vi "VSG25_RampSweep.vi"(0 "Device Handle In":i32, 1 "Run as Subpanel":bool, 2 "RampSweep Cluster In":T1 {"Start Hz" items=["Hz", "kHz", "MHz", "GHz"]; "Stop Hz" items=["Hz", "kHz", "MHz", "GHz"]; "Step Hz" items=["Hz", "kHz", "MHz", "GHz"]}, 3 "Error In":errorcluster) -> (5 "Device Handle Out":i32, 6 "RampSweep Cluster Out":T1 {"Start Hz" items=["Hz", "kHz", "MHz", "GHz"]; "Stop Hz" items=["Hz", "kHz", "MHz", "GHz"]; "Step Hz" items=["Hz", "kHz", "MHz", "GHz"]}, 7 "Error Out":errorcluster)   [LabVIEW 2014]
uses:
  Frequency Hertz.ctl
  RampSweep Cluster.ctl
  sg_lib/VSG25A.lvlib
panel:
  out "Sweep Time":dbl
  out "Frequency Span":dbl
  in  "Dwell Time (mS)":dbl
  in  "Stop":bool
  out "Device Selected":bool
  in  "Step Hz":T2 items=["Hz", "kHz", "MHz", "GHz"]
  in  "Step Frequency":dbl
  in  "Stop Hz":T2 items=["Hz", "kHz", "MHz", "GHz"]
  in  "Stop Frequency":dbl
  in  "RF On":bool
  in  "Start Hz":T2 items=["Hz", "kHz", "MHz", "GHz"]
  in  "Amplitude (dBm)":dbl
  in  "Start Frequency":dbl
  # "Ramp Sweep"
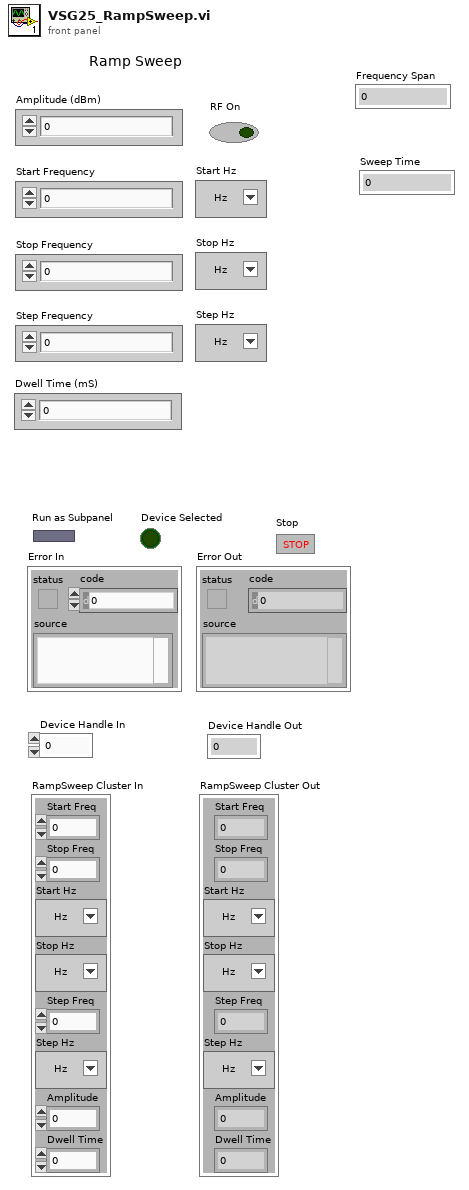
[diagram p1: front panel]
types:
  T1 = typedef "RampSweep Cluster.ctl" = cluster{"Start Freq":dbl, "Stop Freq":dbl, "Start Hz":T2, "Stop Hz":T2, "Step Freq":dbl, "Step Hz":T2, "Amplitude":dbl, "Dwell Time":dbl}
  T2 = typedef "Frequency Hertz.ctl" = u16
  T3 = enum16{"Init", "Proc Events", "Write VSG25", "Exit"}
  T4 = enum32{"Bad", "Idle", "Run top level", "Running"}
  T5 = enum16{"Check Amplitude", "Check Start Freq", "Check Stop Freq", "Check Step Freq", "Check Dwell Time", "Calc Freq Span", "Calc Sweep Time", "Stop RF", "Set Freq And Amp", "Set Sweep", "Finish", ""}
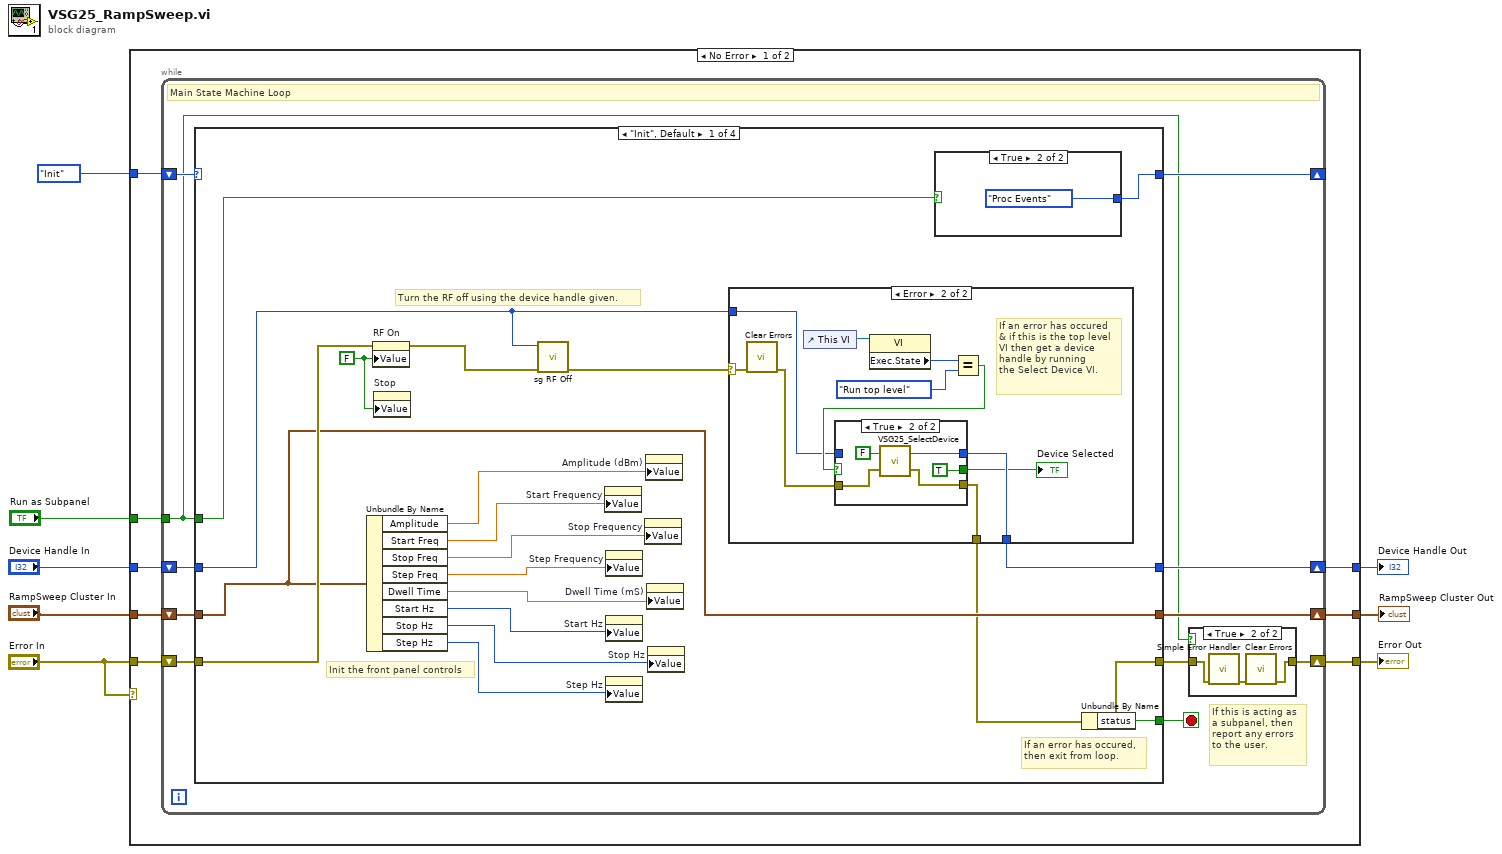
[diagram p0: block diagram]
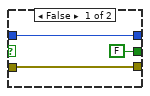
[diagram p4: hidden frame]
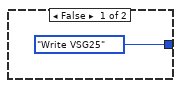
[diagram p5: hidden frame]
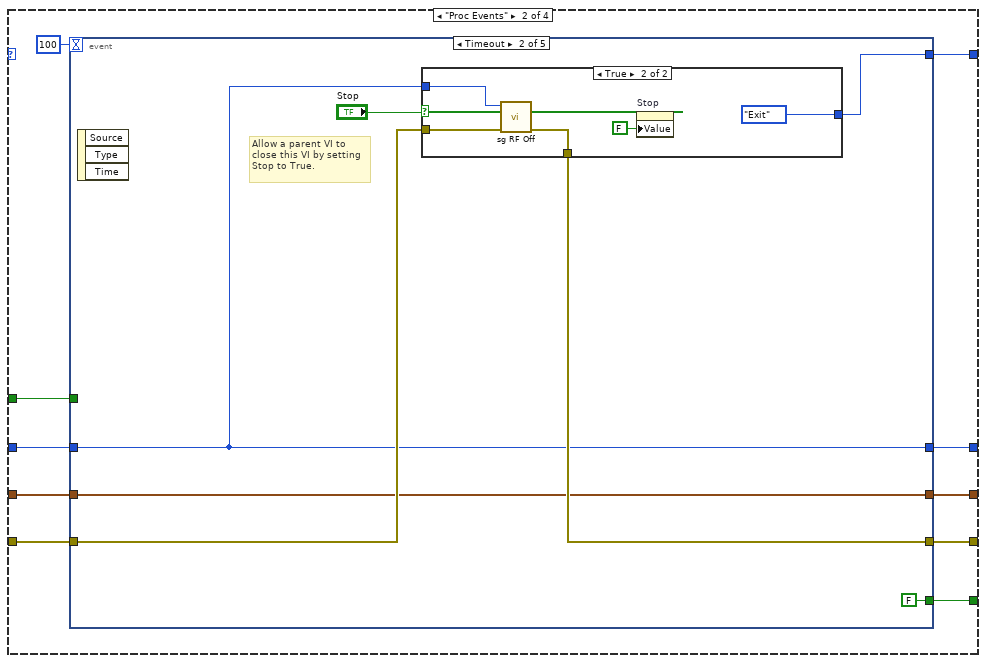
[diagram p6: hidden frame]
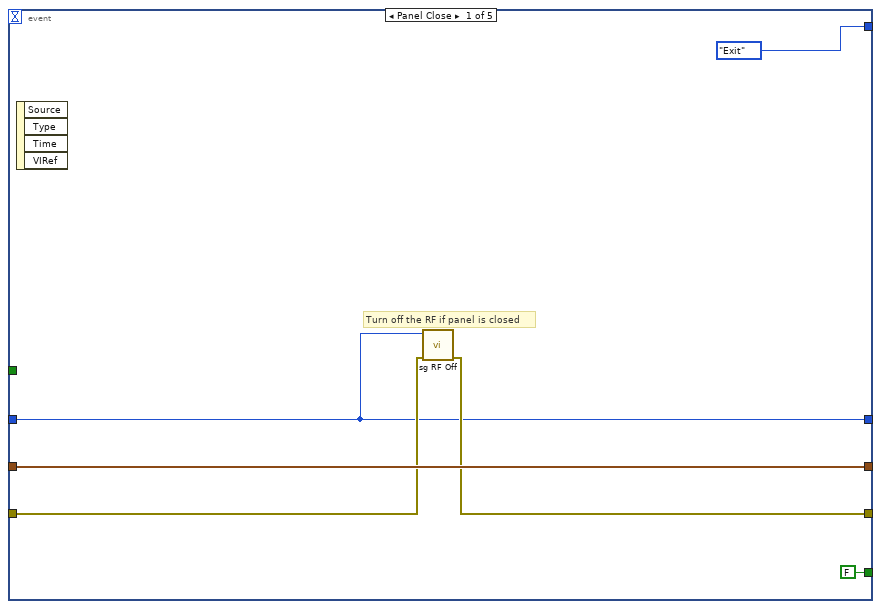
[diagram p7: hidden frame]
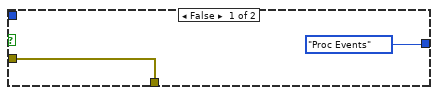
[diagram p8: hidden frame]
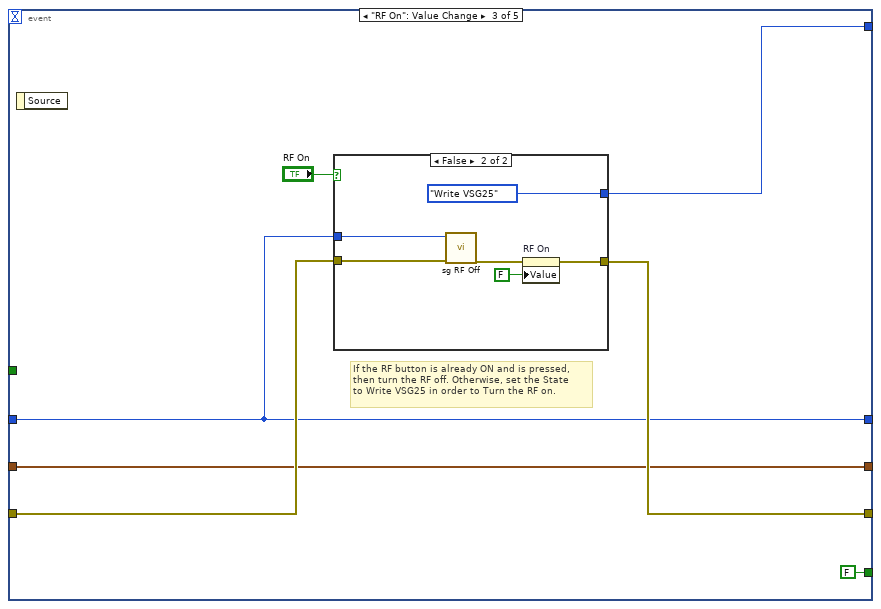
[diagram p9: hidden frame]
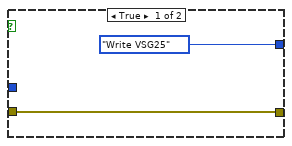
[diagram p10: hidden frame]
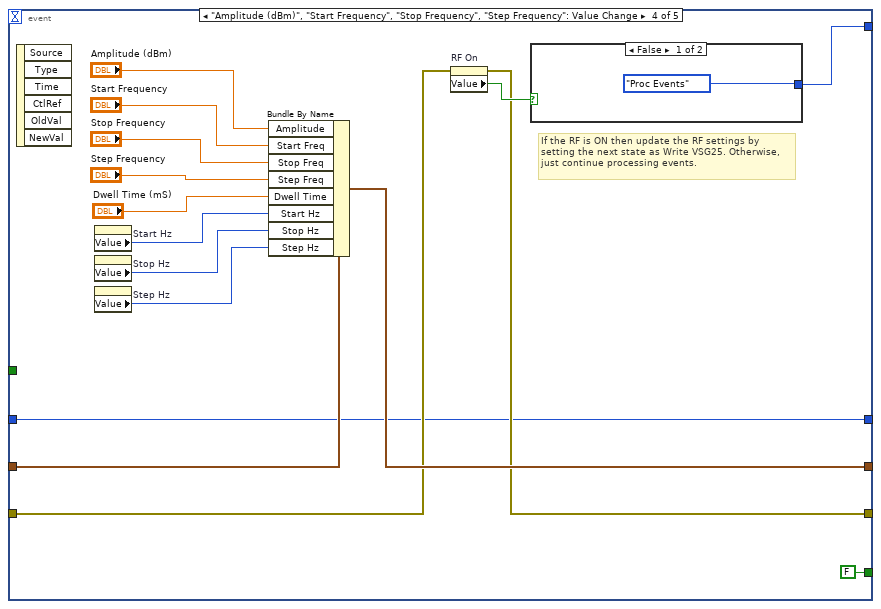
[diagram p11: hidden frame]
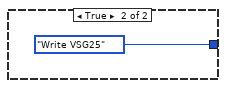
[diagram p12: hidden frame]
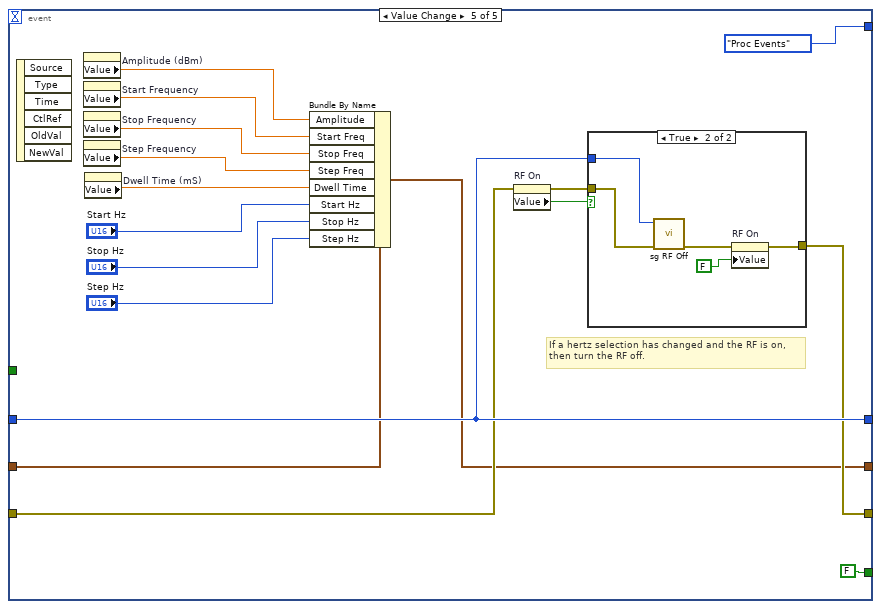
[diagram p13: hidden frame]
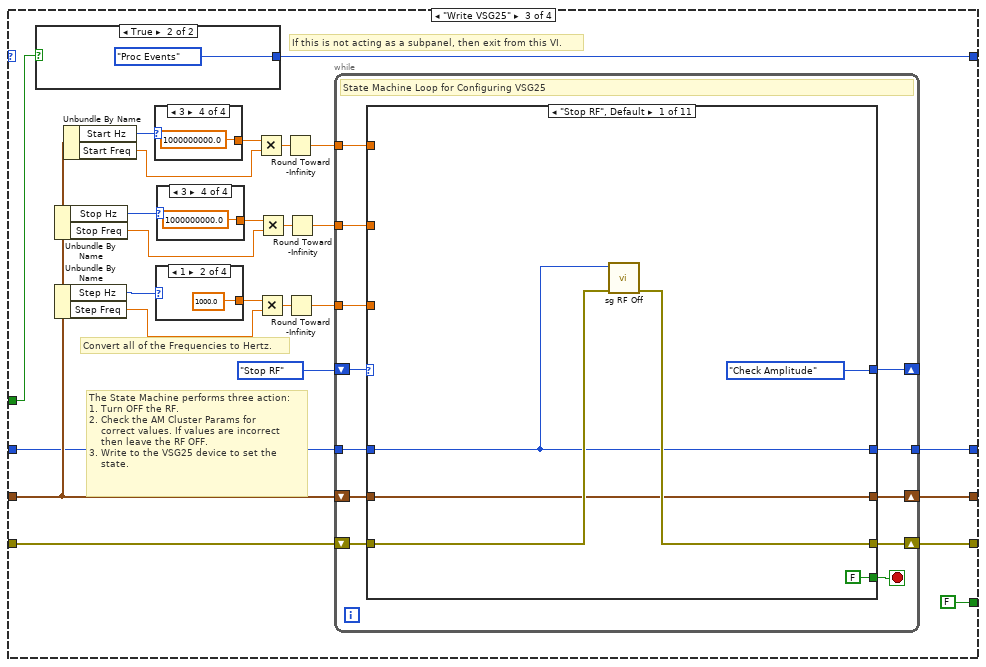
[diagram p15: hidden frame]
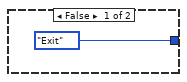
[diagram p16: hidden frame]
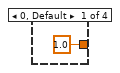
[diagram p17: hidden frame]
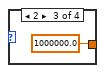
[diagram p18: hidden frame]
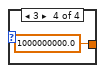
[diagram p19: hidden frame]
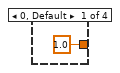
[diagram p20: hidden frame]
diagram:
  n1 = case shown="No Error" "Error In" {
    tunnel: "Error In" -> [w12 w376]
    tunnel: T3."Init" -> [w16 _]
    tunnel: "Run as Subpanel" -> [w15 _]
    tunnel: "Device Handle In" -> [w14 w374]
    tunnel: "RampSweep Cluster In" -> [w13 w375]
    tunnel: [w11 w376] -> w4
    tunnel: [w10 w375] -> w1
    tunnel: [w9 w374] -> w3
    frame No Error {
      n2 = while {
        shift-right: [w26] -> _
        shift-left: w16 -> [w27]
        tunnel: w15 -> [w17]
        shift-right: [w18] -> w11
        shift-left: w12 -> [w23]
        shift-right: [w21] -> w10
        shift-left: w13 -> [w24]
        shift-right: [w20] -> w9
        shift-left: w14 -> [w25]
        stop <- w22 stop-if-true
        # "If this is acting as \na subpanel, then\nreport any errors\nto the user."
        # "Main State Machine Loop"
        n3 = case shown="\"Init\", Default" w27 {
          selector: w27 -> [_ _ _ w369]
          tunnel: [w43 w75 w161 w369] -> w26
          tunnel: w17 -> [w46 w79 w160 _]
          tunnel: w25 -> [w37 w80 w166 w364]
          tunnel: w24 -> [w44 w81 w167 w365]
          tunnel: w23 -> [w45 w82 w171 w366]
          tunnel: [w42 w76 FALSE TRUE] -> w22
          tunnel: [w38 w74 w165 w367] -> w19
          tunnel: [w44 w78 w164 w365] -> w21
          tunnel: [w39 w77 w163 w364] -> w20
          frame "Init", Default {
            w36 = FALSE ("RF On")
            # "Init the front panel controls"
            # "Turn the RF off using the device handle given."
            # "If an error has occured,\nthen exit from loop."
            n4 = Unbundle By Name(w44) -> ("Amplitude"=w50:dbl, "Start Freq"=w49:dbl, "Stop Freq"=w48:dbl, "Step Freq"=w47:dbl, "Dwell Time"=w32:dbl, "Start Hz"=w35:T2, "Stop Hz"=w34:T2, "Step Hz"=w33:T2)
            n5 = property on="RF On" class="Bool (strict)"(error in=w45, "Value"=w36) -> (error out=w41:errorcluster)  [unwired: 1 in, 1 out]
            n6 = property on="Stop" class="Bool (strict)"("Value"=w36) -> ()  [unwired: 2 in, 2 out]
            n7 = call "sg RF Off.vi"("error in (no error)"=w41, "device"=w37) -> ("error out"=w40:errorcluster)  [unwired: 8 in, 1 out]
            n8 = property on="Start Frequency" class="DigNum (strict)"("Value"=w49) -> ()  [unwired: 2 in, 2 out]
            n9 = property on="Step Frequency" class="DigNum (strict)"("Value"=w47) -> ()  [unwired: 2 in, 2 out]
            n10 = property on="Start Hz" class="Ring (strict)"("Value"=w35) -> ()  [unwired: 2 in, 2 out]
            n11 = property on="Step Hz" class="Ring (strict)"("Value"=w33) -> ()  [unwired: 2 in, 2 out]
            n12 = property on="Stop Frequency" class="DigNum (strict)"("Value"=w48) -> ()  [unwired: 2 in, 2 out]
            n13 = property on="Amplitude (dBm)" class="DigNum (strict)"("Value"=w50) -> ()  [unwired: 2 in, 2 out]
            n14 = property on="Dwell Time (mS)" class="DigNum (strict)"("Value"=w32) -> ()  [unwired: 2 in, 2 out]
            n15 = property on="Stop Hz" class="Ring (strict)"("Value"=w34) -> ()  [unwired: 2 in, 2 out]
            n16 = case shown="Error" w40 {
              selector: w40 -> [w51 w58]
              tunnel: [w52 w56] -> w39
              tunnel: [w51 w55] -> w38
              tunnel: w37 -> [w52 w54]
              frame No Error {
              }
              frame Error {
                # "If an error has occured\n& if this is the top level\nVI then get a device\nhandle by running \nthe Select Device VI."
                n17 = call <vilib>:"Clear Errors.vi"("error in (no error)"=w58) -> ("error out"=w57:errorcluster)  [unwired: 5 in, 1 out]
                n18 = control-ref of="This VI"() -> (w62:refnum<vi>)
                n19 = property class="VI"(reference=w62) -> ("Exec.State"=w61:T4)  [unwired: 1 in, 2 out]
                n20 = Equal?(x=w61, y=T4."Run top level" ("Execution:State 2")) -> (x = y?=w59:bool)
                n21 = case shown="True" w59 {
                  tunnel: [w65 w70] -> w56
                  tunnel: w54 -> [w65 _]
                  tunnel: w57 -> [w64 w68]
                  tunnel: [w64 w67] -> w55
                  tunnel: [FALSE TRUE] -> w53
                  frame False {
                  }
                  frame True {
                    n22 = call "VSG25_SelectDevice.vi"("ErrorIn"=w68, "AutoSel"=FALSE) -> ("ErrorOut"=w67:errorcluster, "deviceHandle"=w70:i32)
                  }
                }
                "Device Selected" <- w53
              }
            }
            n23 = case shown="True" w46 {
              tunnel: [T3."Write VSG25" T3."Proc Events"] -> w43
              frame False {
              }
              frame True {
              }
            }
            n24 = Unbundle By Name(w38) -> ("status"=w42:bool)
          }
          frame "Proc Events" {
            n25 = event shown="[1] Timeout" {
              selector: _ -> [_ _ _ _ _]
              dyn-events: _ -> [_ _ _ _ _]
              timeout: 100 -> [_ _ _ _ _]
              tunnel: w82 -> [w85 w92 w108 w125 w148]
              tunnel: w81 -> [w86 w90 w106 w133 w147]
              tunnel: w80 -> [w83 w89 w105 w123 w150]
              tunnel: w79 -> [_ _ _ _ _]
              tunnel: [w84 w91 w107 w124 w149] -> w74
              tunnel: [w86 w90 w106 w132 w146] -> w78
              tunnel: [w83 w89 w105 w123 w150] -> w77
              tunnel: [FALSE FALSE FALSE FALSE FALSE] -> w76
              tunnel: [T3."Exit" w93 w104 w126 T3."Proc Events"] -> w75
              event Panel Close {
                # "Turn off the RF if panel is closed"
                n26 = event-data() -> ()  [unwired: 1 in, 4 out]
                n27 = call "sg RF Off.vi"("error in (no error)"=w85, "device"=w83) -> ("error out"=w84:errorcluster)  [unwired: 8 in, 1 out]
              }
              event Timeout {
                # "Allow a parent VI to \nclose this VI by setting\nStop to True."
                n28 = event-data() -> ()  [unwired: 1 in, 3 out]
                n29 = case shown="True" "Stop" {
                  tunnel: [T3."Proc Events" T3."Exit"] -> w93
                  tunnel: w92 -> [w96 w101]
                  tunnel: [w96 w100] -> w91
                  tunnel: w89 -> [_ w99]
                  frame False {
                  }
                  frame True {
                    n30 = call "sg RF Off.vi"("error in (no error)"=w101, "device"=w99) -> ("error out"=w100:errorcluster)  [unwired: 8 in, 1 out]
                    n31 = property on="Stop" class="Bool (strict)"("Value"=FALSE ("Stop")) -> ()  [unwired: 2 in, 2 out]
                  }
                }
              }
              event "RF On": Value Change {
                # "If the RF button is already ON and is pressed, \nthen turn the RF off. Otherwise, set the State\nto Write VSG25 in order to Turn the RF on."
                n32 = event-data() -> ()  [unwired: 1 in, 1 out]
                n33 = case shown="False" "RF On" {
                  tunnel: [w110 w115] -> w107
                  tunnel: w108 -> [w110 w117]
                  tunnel: w105 -> [_ w116]
                  tunnel: [T3."Write VSG25" T3."Write VSG25"] -> w104
                  frame True {
                  }
                  frame False {
                    n34 = call "sg RF Off.vi"("error in (no error)"=w117, "device"=w116) -> ("error out"=w114:errorcluster)  [unwired: 8 in, 1 out]
                    n35 = property on="RF On" class="Bool (strict)"(error in=w114, "Value"=FALSE ("RF On")) -> (error out=w115:errorcluster)  [unwired: 1 in, 1 out]
                  }
                }
              }
              event "Amplitude (dBm)", "Start Frequency", "Stop Frequency", "Step Frequency": Value Change {
                # "If the RF is ON then update the RF settings by\nsetting the next state as Write VSG25. Otherwise,\njust continue processing events."
                n36 = event-data() -> ()  [unwired: 1 in, 6 out]
                n37 = property on="Start Hz" class="Ring (strict)"() -> ("Value"=w120:T2)  [unwired: 2 in, 2 out]
                n38 = property on="Stop Hz" class="Ring (strict)"() -> ("Value"=w119:T2)  [unwired: 2 in, 2 out]
                n39 = property on="Step Hz" class="Ring (strict)"() -> ("Value"=w118:T2)  [unwired: 2 in, 2 out]
                n40 = Bundle By Name(cluster=w133, "Amplitude"="Amplitude (dBm)", "Start Freq"="Start Frequency", "Stop Freq"="Stop Frequency", "Step Freq"="Step Frequency", "Dwell Time"="Dwell Time (mS)", "Start Hz"=w120, "Stop Hz"=w119, "Step Hz"=w118) -> (w132:T1)
                n41 = property on="RF On" class="Bool (strict)"(error in=w125) -> (error out=w124:errorcluster, "Value"=w127:bool)  [unwired: 1 in, 1 out]
                n42 = case shown="False" w127 {
                  tunnel: [T3."Proc Events" T3."Write VSG25"] -> w126
                  frame False {
                  }
                  frame True {
                  }
                }
              }
              event Value Change {
                # "If a hertz selection has changed and the RF is on,\nthen turn the RF off."
                n43 = event-data() -> ()  [unwired: 1 in, 6 out]
                n44 = property on="Amplitude (dBm)" class="DigNum (strict)"() -> ("Value"=w145:dbl)  [unwired: 2 in, 2 out]
                n45 = property on="Start Frequency" class="DigNum (strict)"() -> ("Value"=w144:dbl)  [unwired: 2 in, 2 out]
                n46 = property on="Stop Frequency" class="DigNum (strict)"() -> ("Value"=w143:dbl)  [unwired: 2 in, 2 out]
                n47 = property on="Step Frequency" class="DigNum (strict)"() -> ("Value"=w142:dbl)  [unwired: 2 in, 2 out]
                n48 = property on="Dwell Time (mS)" class="DigNum (strict)"() -> ("Value"=w139:dbl)  [unwired: 2 in, 2 out]
                n49 = Bundle By Name(cluster=w147, "Amplitude"=w145, "Start Freq"=w144, "Stop Freq"=w143, "Step Freq"=w142, "Dwell Time"=w139, "Start Hz"="Start Hz", "Stop Hz"="Stop Hz", "Step Hz"="Step Hz") -> (w146:T1)
                n50 = property on="RF On" class="Bool (strict)"(error in=w148) -> (error out=w152:errorcluster, "Value"=w151:bool)  [unwired: 1 in, 1 out]
                n51 = case shown="True" w151 {
                  tunnel: [w153 w154] -> w149
                  tunnel: w152 -> [w153 w158]
                  tunnel: w150 -> [_ w157]
                  frame False {
                  }
                  frame True {
                    n52 = call "sg RF Off.vi"("error in (no error)"=w158, "device"=w157) -> ("error out"=w155:errorcluster)  [unwired: 8 in, 1 out]
                    n53 = property on="RF On" class="Bool (strict)"(error in=w155, "Value"=FALSE ("RF On")) -> (error out=w154:errorcluster)  [unwired: 1 in, 1 out]
                  }
                }
              }
            }
          }
          frame "Write VSG25" {
            # "If this is not acting as a subpanel, then exit from this VI."
            # "Convert all of the Frequencies to Hertz."
            # "The State Machine performs three action:\n1. Turn OFF the RF.\n2. Check the AM Cluster Params for \n    correct values. If values are incorrect\n    then leave the RF OFF.\n3. Write to the VSG25 device to set the\n    state."
            n54 = case shown="True" w160 {
              tunnel: [T3."Exit" T3."Proc Events"] -> w161
              frame False {
              }
              frame True {
              }
            }
            n55 = Unbundle By Name(w167) -> ("Stop Hz"=w177:T2, "Stop Freq"=w179:dbl)
            n56 = Unbundle By Name(w167) -> ("Step Hz"=w173:T2, "Step Freq"=w175:dbl)
            n57 = Unbundle By Name(w167) -> ("Start Hz"=w182:T2, "Start Freq"=w180:dbl)
            n58 = case shown="3" w182 {
              tunnel: [1.0 ("y") 1000.0 ("y") 1000000.0 ("y") 1000000000.0 ("y")] -> w181
              frame 0, Default {
              }
              frame 1 {
              }
              frame 2 {
              }
              frame 3 {
              }
            }
            n59 = case shown="1" w173 {
              tunnel: [1.0 ("y") 1000.0 ("y") 1000000.0 ("y") 1000000000.0 ("y")] -> w174
              frame 0, Default {
              }
              frame 1 {
              }
              frame 2 {
              }
              frame 3 {
              }
            }
            n60 = case shown="3" w177 {
              tunnel: [1.0 ("y") 1000.0 ("y") 1000000.0 ("y") 1000000000.0 ("y")] -> w178
              frame 0, Default {
              }
              frame 1 {
              }
              frame 2 {
              }
              frame 3 {
              }
            }
            n61 = Multiply(x=w181, y=w180) -> (x*y=w183:dbl)
            n62 = Multiply(x=w174, y=w175) -> (x*y=w172:dbl)
            n63 = Multiply(x=w178, y=w179) -> (x*y=w176:dbl)
            n64 = Round Toward -Infinity(1:w183) -> (0:w170:dbl)
            n65 = Round Toward -Infinity(1:w172) -> (0:w168:dbl)
            n66 = Round Toward -Infinity(1:w176) -> (0:w169:dbl)
            n67 = while {
              shift-right: [w194] -> _
              shift-left: T5."Stop RF" -> [w205]
              tunnel: w170 -> [w203]
              tunnel: w169 -> [w202]
              tunnel: w168 -> [w201]
              tunnel: w166 -> [w199]
              tunnel: [w196] -> w163
              shift-right: [w198] -> w165
              shift-left: w171 -> [w204]
              shift-right: [w197] -> w164
              shift-left: w167 -> [w200]
              stop <- w195 stop-if-true
              # "State Machine Loop for Configuring VSG25"
              n68 = case shown="\"Stop RF\", Default" w205 {
                selector: w205 -> [_ _ _ _ _ _ _ _ _ _ w354]
                tunnel: w204 -> [w211 w214 w252 w270 w288 w305 w317 w322 w340 w349 w351]
                tunnel: w203 -> [_ _ w242 _ _ _ w315 _ w332 _ _]
                tunnel: w202 -> [_ _ w244 w264 _ _ w314 _ _ _ _]
                tunnel: w201 -> [_ _ w243 _ w282 _ _ _ _ _ _]
                tunnel: w200 -> [w209 w218 w253 w272 w290 w303 w321 w323 w338 w347 w352]
                tunnel: w199 -> [w208 w216 w254 w271 w289 w302 w320 w330 w337 w346 w353]
                tunnel: [w210 w213 w251 w269 w287 w304 w317 w322 w339 w348 w351] -> w198
                tunnel: [w209 w217 w253 w272 w290 w303 w321 w323 w338 w347 w352] -> w197
                tunnel: [w208 w216 w254 w271 w289 w302 w320 w330 w337 w346 w353] -> w196
                tunnel: [FALSE FALSE FALSE FALSE FALSE FALSE FALSE FALSE FALSE FALSE TRUE] -> w195
                tunnel: [T5."Check Amplitude" w212 w256 w274 w292 w299 T5."Calc Sweep Time" T5."Set Freq And Amp" T5."Set Sweep" T5."Finish" w354] -> w194
                frame "Stop RF", Default {
                  n69 = call "sg RF Off.vi"("error in (no error)"=w211, "device"=w208) -> ("error out"=w210:errorcluster)  [unwired: 8 in, 1 out]
                }
                frame "Check Amplitude" {
                  n70 = Unbundle By Name(w218) -> ("Amplitude"=w224:dbl)
                  n71 = Less Or Equal?(x=w224, y=10.0) -> (x <= y?=w220:bool)
                  n72 = Greater Or Equal?(x=w224, y=-80.0) -> (x >= y?=w223:bool)
                  n73 = And(x=w220, y=w223) -> (x .and. y?=w219:bool)
                  n74 = case shown="True" w219 {
                    tunnel: w223 -> [w234 _]
                    tunnel: w224 -> [_ w239]
                    tunnel: w218 -> [w231 w238]
                    tunnel: [w230 w237] -> w217
                    tunnel: [T5."Finish" T5."Check Start Freq"] -> w212
                    tunnel: w214 -> [w228 w236]
                    tunnel: [w226 w236] -> w213
                    frame False {
                      n75 = Select(t=10.0, s=w234, f=-80.0) -> (s? t:f=w229:dbl)
                      n76 = Bundle By Name(cluster=w231, "Start Freq"=w229) -> (w230:T1)
                      n77 = property on="Amplitude (dBm)" class="DigNum (strict)"("Value"=w229) -> ()  [unwired: 2 in, 2 out]
                      n78 = Merge Errors(w228, errorcluster {"status"=TRUE, "code"=-1, "source"="Invalid Amplitude.\nValue must be between\n-80 dBm and 10 dBm."} ("error constant")) -> (w226:errorcluster)
                    }
                    frame True {
                      n79 = Round Toward -Infinity(1:w239) -> (0:w240:dbl)
                      n80 = Bundle By Name(cluster=w238, "Amplitude"=w240) -> (w237:T1)
                    }
                  }
                }
                frame "Check Start Freq" {
                  n81 = Subtract(x=w244, y=w243) -> (x-y=w246:dbl)
                  n82 = Greater Or Equal?(x=w242, y=80000000.0) -> (x >= y?=w248:bool)
                  n83 = Less Or Equal?(x=w242, y=w246) -> (x <= y?=w249:bool)
                  n84 = Less Or Equal?(x=w242, y=2500000000.0) -> (x <= y?=w250:bool)
                  n85 = Compound Arithmetic op=AND(w248, w249, w250) -> (w241:bool)
                  n86 = case shown="False" w241 {
                    tunnel: [T5."Finish" T5."Check Stop Freq"] -> w256
                    tunnel: w252 -> [w259 w262]
                    tunnel: [w260 w262] -> w251
                    frame False {
                      n87 = Merge Errors(w259, errorcluster {"status"=TRUE, "code"=-1, "source"="Start frequency must \nbe greater than 80 MHz,\nless than 2.5 GHz and \nless than stop frequency \nby one step."} ("error constant")) -> (w260:errorcluster)
                    }
                    frame True {
                    }
                  }
                }
                frame "Check Stop Freq" {
                  n88 = Greater Or Equal?(x=w264, y=80000000.0) -> (x >= y?=w267:bool)
                  n89 = Less Or Equal?(x=w264, y=2500000000.0) -> (x <= y?=w268:bool)
                  n90 = Compound Arithmetic op=AND(w267, w268) -> (w263:bool)
                  n91 = case shown="False" w263 {
                    tunnel: [T5."Finish" T5."Check Step Freq"] -> w274
                    tunnel: w270 -> [w278 w280]
                    tunnel: [w276 w280] -> w269
                    frame False {
                      n92 = Merge Errors(w278, errorcluster {"status"=TRUE, "code"=-1, "source"="Stop frequency must \nbe greater than 80 MHz,\nand less than 2.5 GHz."} ("error constant")) -> (w276:errorcluster)
                    }
                    frame True {
                    }
                  }
                }
                frame "Check Step Freq" {
                  n93 = Greater Or Equal?(x=w282, y=80000000.0) -> (x >= y?=w285:bool)
                  n94 = Less Or Equal?(x=w282, y=2500000000.0) -> (x <= y?=w286:bool)
                  n95 = Compound Arithmetic op=AND(w285, w286) -> (w281:bool)
                  n96 = case shown="False" w281 {
                    tunnel: [T5."Finish" T5."Check Dwell Time"] -> w292
                    tunnel: w288 -> [w295 w298]
                    tunnel: [w296 w298] -> w287
                    frame False {
                      n97 = Merge Errors(w295, errorcluster {"status"=TRUE, "code"=-1, "source"="Step frequency must \nbe greater than 80 MHz,\nand less than 2.5 GHz."} ("error constant")) -> (w296:errorcluster)
                    }
                    frame True {
                    }
                  }
                }
                frame "Check Dwell Time" {
                  n98 = Unbundle By Name(w303) -> ("Dwell Time"=w306:dbl)
                  n99 = Greater Or Equal?(x=w306, y=1.0) -> (x >= y?=w301:bool)
                  n100 = case shown="False" w301 {
                    tunnel: [T5."Finish" T5."Calc Freq Span"] -> w299
                    tunnel: w305 -> [w310 w313]
                    tunnel: [w311 w313] -> w304
                    frame False {
                      n101 = Merge Errors(w310, errorcluster {"status"=TRUE, "code"=-1, "source"="Dwell time must be greater \nthan 1 milliSecond."} ("error constant")) -> (w311:errorcluster)
                    }
                    frame True {
                    }
                  }
                }
                frame "Calc Freq Span" {
                  n102 = Subtract(x=w314, y=w315) -> (x-y=→"Frequency Span":dbl)
                }
                frame "Calc Sweep Time" {
                  n103 = Unbundle By Name(w323) -> ("Dwell Time"=w326:dbl)
                  n104 = Divide(x=w326, y=1000.0) -> (x/y=w328:dbl)
                  n105 = Round Toward -Infinity(1:w328) -> (0:→"Sweep Time":dbl)
                }
                frame "Set Freq And Amp" {
                  n106 = property on="Frequency Span" class="DigNum (strict)"() -> ("Value"=w333:dbl)  [unwired: 2 in, 2 out]
                  n107 = Divide(x=w333, y=2.0) -> (x/y=w335:dbl)
                  n108 = Unbundle By Name(w338) -> ("Amplitude"=w342:dbl)
                  n109 = Add(x=w332, y=w335) -> (x+y=w331:dbl)
                  n110 = call "sg Set Frequency Amplitude.vi"("error in (no error)"=w340, "amplitude"=w342, "frequency"=w331, "device"=w337) -> ("error out"=w339:errorcluster)  [unwired: 6 in, 1 out]
                }
                frame "Set Sweep" {
                  n111 = property on="Frequency Span" class="DigNum (strict)"() -> ("Value"=w344:dbl)  [unwired: 2 in, 2 out]
                  n112 = property on="Sweep Time" class="DigNum (strict)"() -> ("Value"=w343:dbl)  [unwired: 2 in, 2 out]
                  n113 = call "sg Set Sweep.vi"("error in (no error)"=w349, "span"=w343, "time"=w344, "device"=w346) -> ("error out"=w348:errorcluster)  [unwired: 6 in, 1 out]
                }
                frame "Finish" {
                  # "If no errors have occured, then indicate that the RF is ON."
                  n114 = case shown="Error" w351 {
                    tunnel: [TRUE FALSE] -> w356
                    frame No Error {
                    }
                    frame Error {
                    }
                  }
                  n115 = property on="RF On" class="Bool (strict)"("Value"=w356) -> ()  [unwired: 2 in, 2 out]
                }
              }
            }
          }
          frame "Exit" {
            # "If a device handle was\nacquired using the \nSelect Device VI, then\nclose the handle \nbefore exiting."
            n116 = local read "Device Selected"() -> (w363:bool)
            n117 = case shown="True" w363 {
              tunnel: w364 -> [_ w373]
              tunnel: w366 -> [w370 w372]
              tunnel: [w370 w371] -> w367
              frame False {
              }
              frame True {
                n118 = call "sg Close Device.vi"("error in (no error)"=w372, "device"=w373) -> ("error out"=w371:errorcluster)  [unwired: 8 in, 1 out]
              }
            }
          }
        }
        n119 = case shown="True" w17 {
          tunnel: w19 -> [w28 w30]
          tunnel: [w28 w31] -> w18
          frame False {
          }
          frame True {
            n120 = call <vilib>:"Simple Error Handler.vi"("error in (no error)"=w30) -> ("error out"=w29:errorcluster)  [unwired: 4 in, 4 out]
            n121 = call <vilib>:"Clear Errors.vi"("error in (no error)"=w29) -> ("error out"=w31:errorcluster)  [unwired: 5 in, 1 out]
          }
        }
      }
    }
    frame Error {
    }
  }
  "Error Out" <- w4
  "Device Handle Out" <- w3
  "RampSweep Cluster Out" <- w1
